vi "Get Events.vi"(11 "Test Channel View in":refnum<class "Test Channel View.lvclass">) -> (2 "Events":T1, 3 "Test Channel View out":refnum<class "Test Channel View.lvclass">)   [LabVIEW 2013, in "Test Channel View.lvlib" / "Test Channel View.lvclass"]
uses:
  Test Channel View.lvclass
  Typedef/Events.ctl
  Test Channel View.lvclass/Test Channel View.ctl
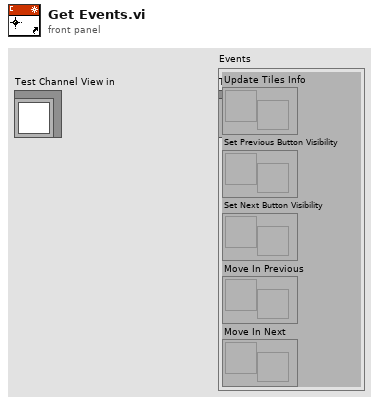
[diagram p1: front panel]
types:
  T1 = typedef "Test Channel View.lvlib/Test Channel View.lvclass/Events.ctl" = cluster{"Update Tiles Info":refnum<user-event>, "Set Previous Button Visibility":refnum<user-event>, "Set Next Button Visibility":refnum<user-event>, "Move In Previous":refnum<user-event>, "Move In Next":refnum<user-event>}
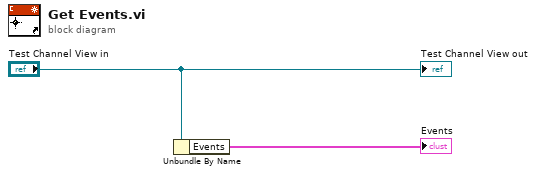
[diagram p0: block diagram]
diagram:
  n1 = Unbundle By Name("Test Channel View in") -> ("Events"=→"Events":T1)
  "Test Channel View out" <- "Test Channel View in"
